vi "Lookup Implementor.vi"(8 "error in (no error)":errorcluster, 10 "Implementor ID":string, 11 "Data in":T1) -> (0 "error out":errorcluster, 1 "Found?":bool, 3 "Data out":T1)   [LabVIEW 2020, in "Peek Window.lvlib"]
uses:
  Peek Window.lvlib
  MHL Data Cluster.ctl
  Standard VI Type/Standard VI Type.lvclass
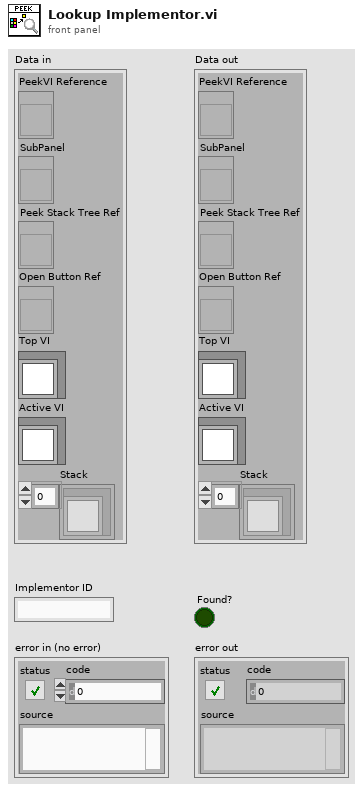
[diagram p1: front panel]
types:
  T1 = typedef "Peek Window.lvlib/MHL Data Cluster.ctl" = cluster{"PeekVI Reference":refnum<vi>, "SubPanel":refnum<vi>, "Peek Stack Tree Ref":refnum<vi>, "Open Button Ref":refnum<vi>, "Top VI":refnum<class "Standard VI Type.lvclass">, "Active VI":refnum<class "Standard VI Type.lvclass">, "Stack":refnum<class "Standard VI Type.lvclass">[]}
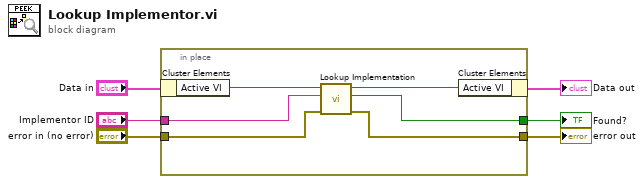
[diagram p0: block diagram]
diagram:
  n1 = in-place {
    in-place-border: "Implementor ID" -> [w12]
    in-place-border: [w11] -> w1
    in-place-border: "error in (no error)" -> [w8]
    in-place-border: [w7] -> w2
    n2 = in-place-cluster #1("Data in") -> ("Active VI"=w10:refnum<class "Standard VI Type.lvclass">)
    n3 = call-dynamic "Lookup Implementation.vi"("error in (no error)"=w8, "Implementation Tag"=w12, "Standard VI Type in"=w10) -> ("error out"=w7:errorcluster, "Found?"=w11:bool, "Standard VI Type out"=w9:refnum<class "Standard VI Type.lvclass">)  [unwired: 6 in]
    n4 = in-place-cluster #1("Active VI"=w9) -> (→"Data out":T1)
  }
  "error out" <- w2
  "Found?" <- w1
